vi "test.vi"() -> ()   [LabVIEW 2016]
uses:
  C:/Users/sciollalab/Documents/Brandeis-BNL/LabVIEW_Codes/BNLStaveAssembly-Blueprint/Bin/Aerotech.A3200.dll
  BNLStaveAssembly-Blueprint/Bin/Aerotech.A3200.dll
panel:
  in  "Axis Speeds":T1={"X [mm/s]"=10.0, "Y [mm/s]"=10.0, "Z [mm/s]"=10.0}
  out "Moving":bool
  in  "Program Errors":errorcluster
  out "XYZ Stage Control":refnum<k24>
  out "Stave origin":T2
  in  "XYZ Stage Frame: Coordinates for calibration":T3={"Stave origin"={"X [mm]"=-706.0, "Y [mm]"=140.5, "Z [mm]"=-13.5}, "Autofocus"={"X [mm]"=-686.0, "Y [mm]"=130.0, "Z [mm]"=-18.0}, "Calib Pattern"={"X [mm]"=-566.0, "Y [mm]"=39.26, "Z [mm]"=-22.0}}
  out "Current stage position [mm]":cluster{"X":dbl, "Y":dbl, "Z":dbl}
  in  "Update jog increment":bool
  in  "Jog step size":T2={"X [mm]"=0.1, "Y [mm]"=0.1, "Z [mm]"=0.1}
  in  "Backward":bool
  in  "Reset position":bool
  in  "Left":bool
  in  "Right":bool
  in  "Confirm position":bool
  in  "Forward":bool
  out "element":string
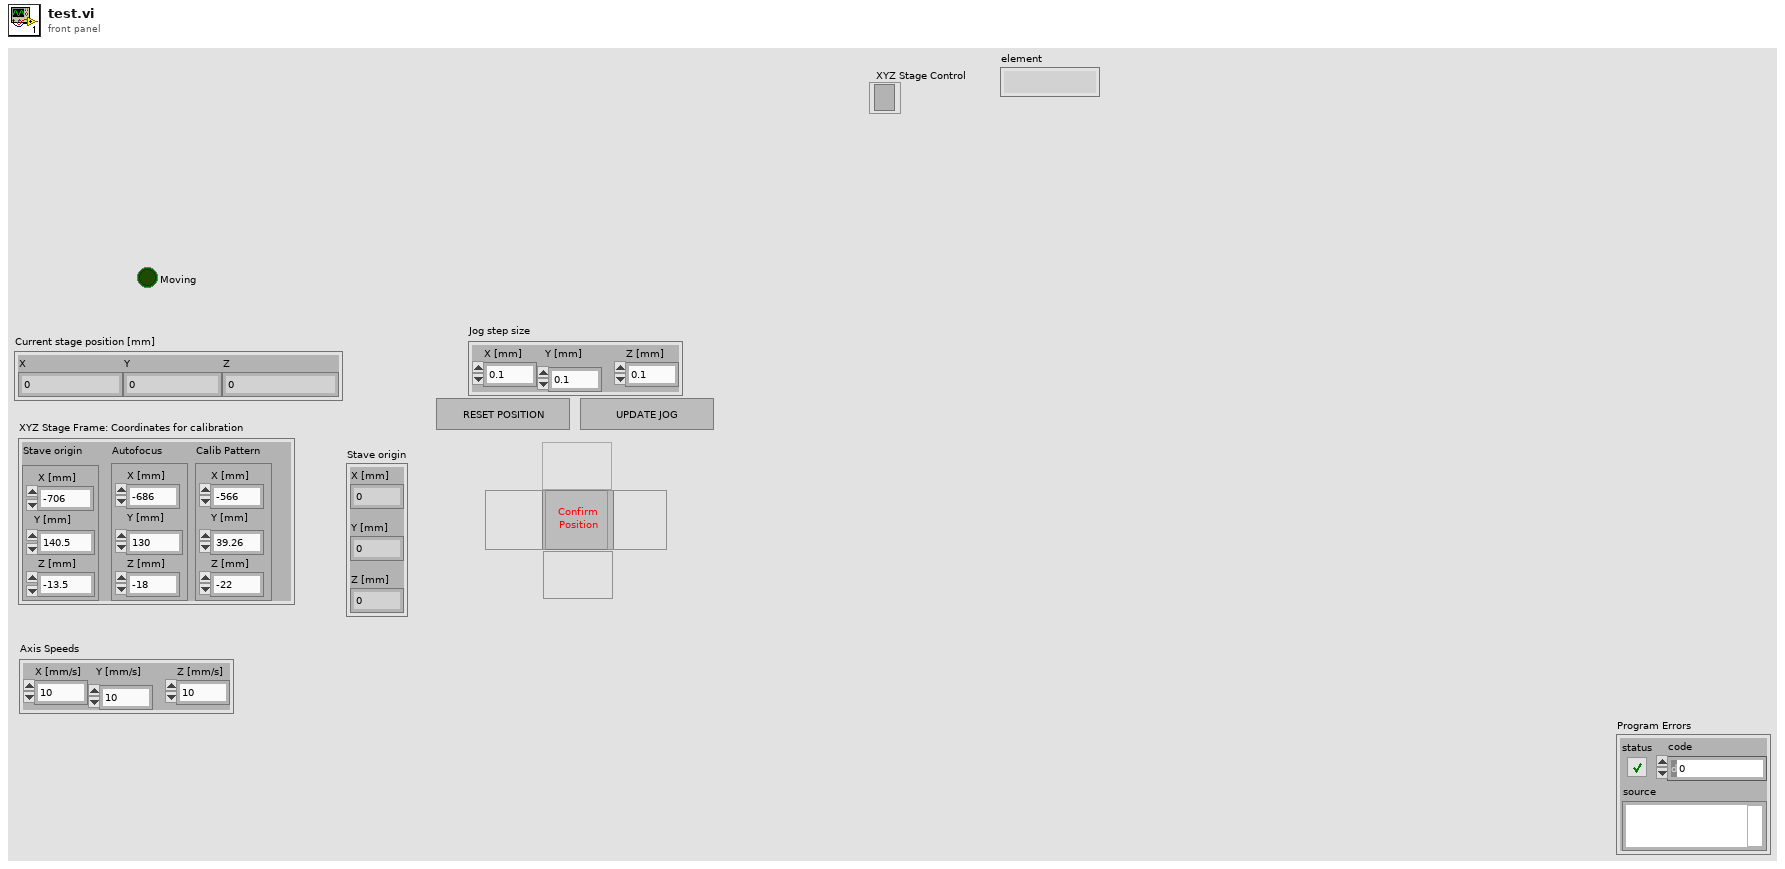
[diagram p1: front panel]
types:
  T1 = cluster{"X [mm/s]":dbl, "Y [mm/s]":dbl, "Z [mm/s]":dbl}
  T2 = cluster{"X [mm]":dbl, "Y [mm]":dbl, "Z [mm]":dbl}
  T3 = cluster{"Stave origin":cluster{"X [mm]":dbl, "Y [mm]":dbl, "Z [mm]":dbl}, "Autofocus":cluster{"X [mm]":dbl, "Y [mm]":dbl, "Z [mm]":dbl}, "Calib Pattern":cluster{"X [mm]":dbl, "Y [mm]":dbl, "Z [mm]":dbl}}
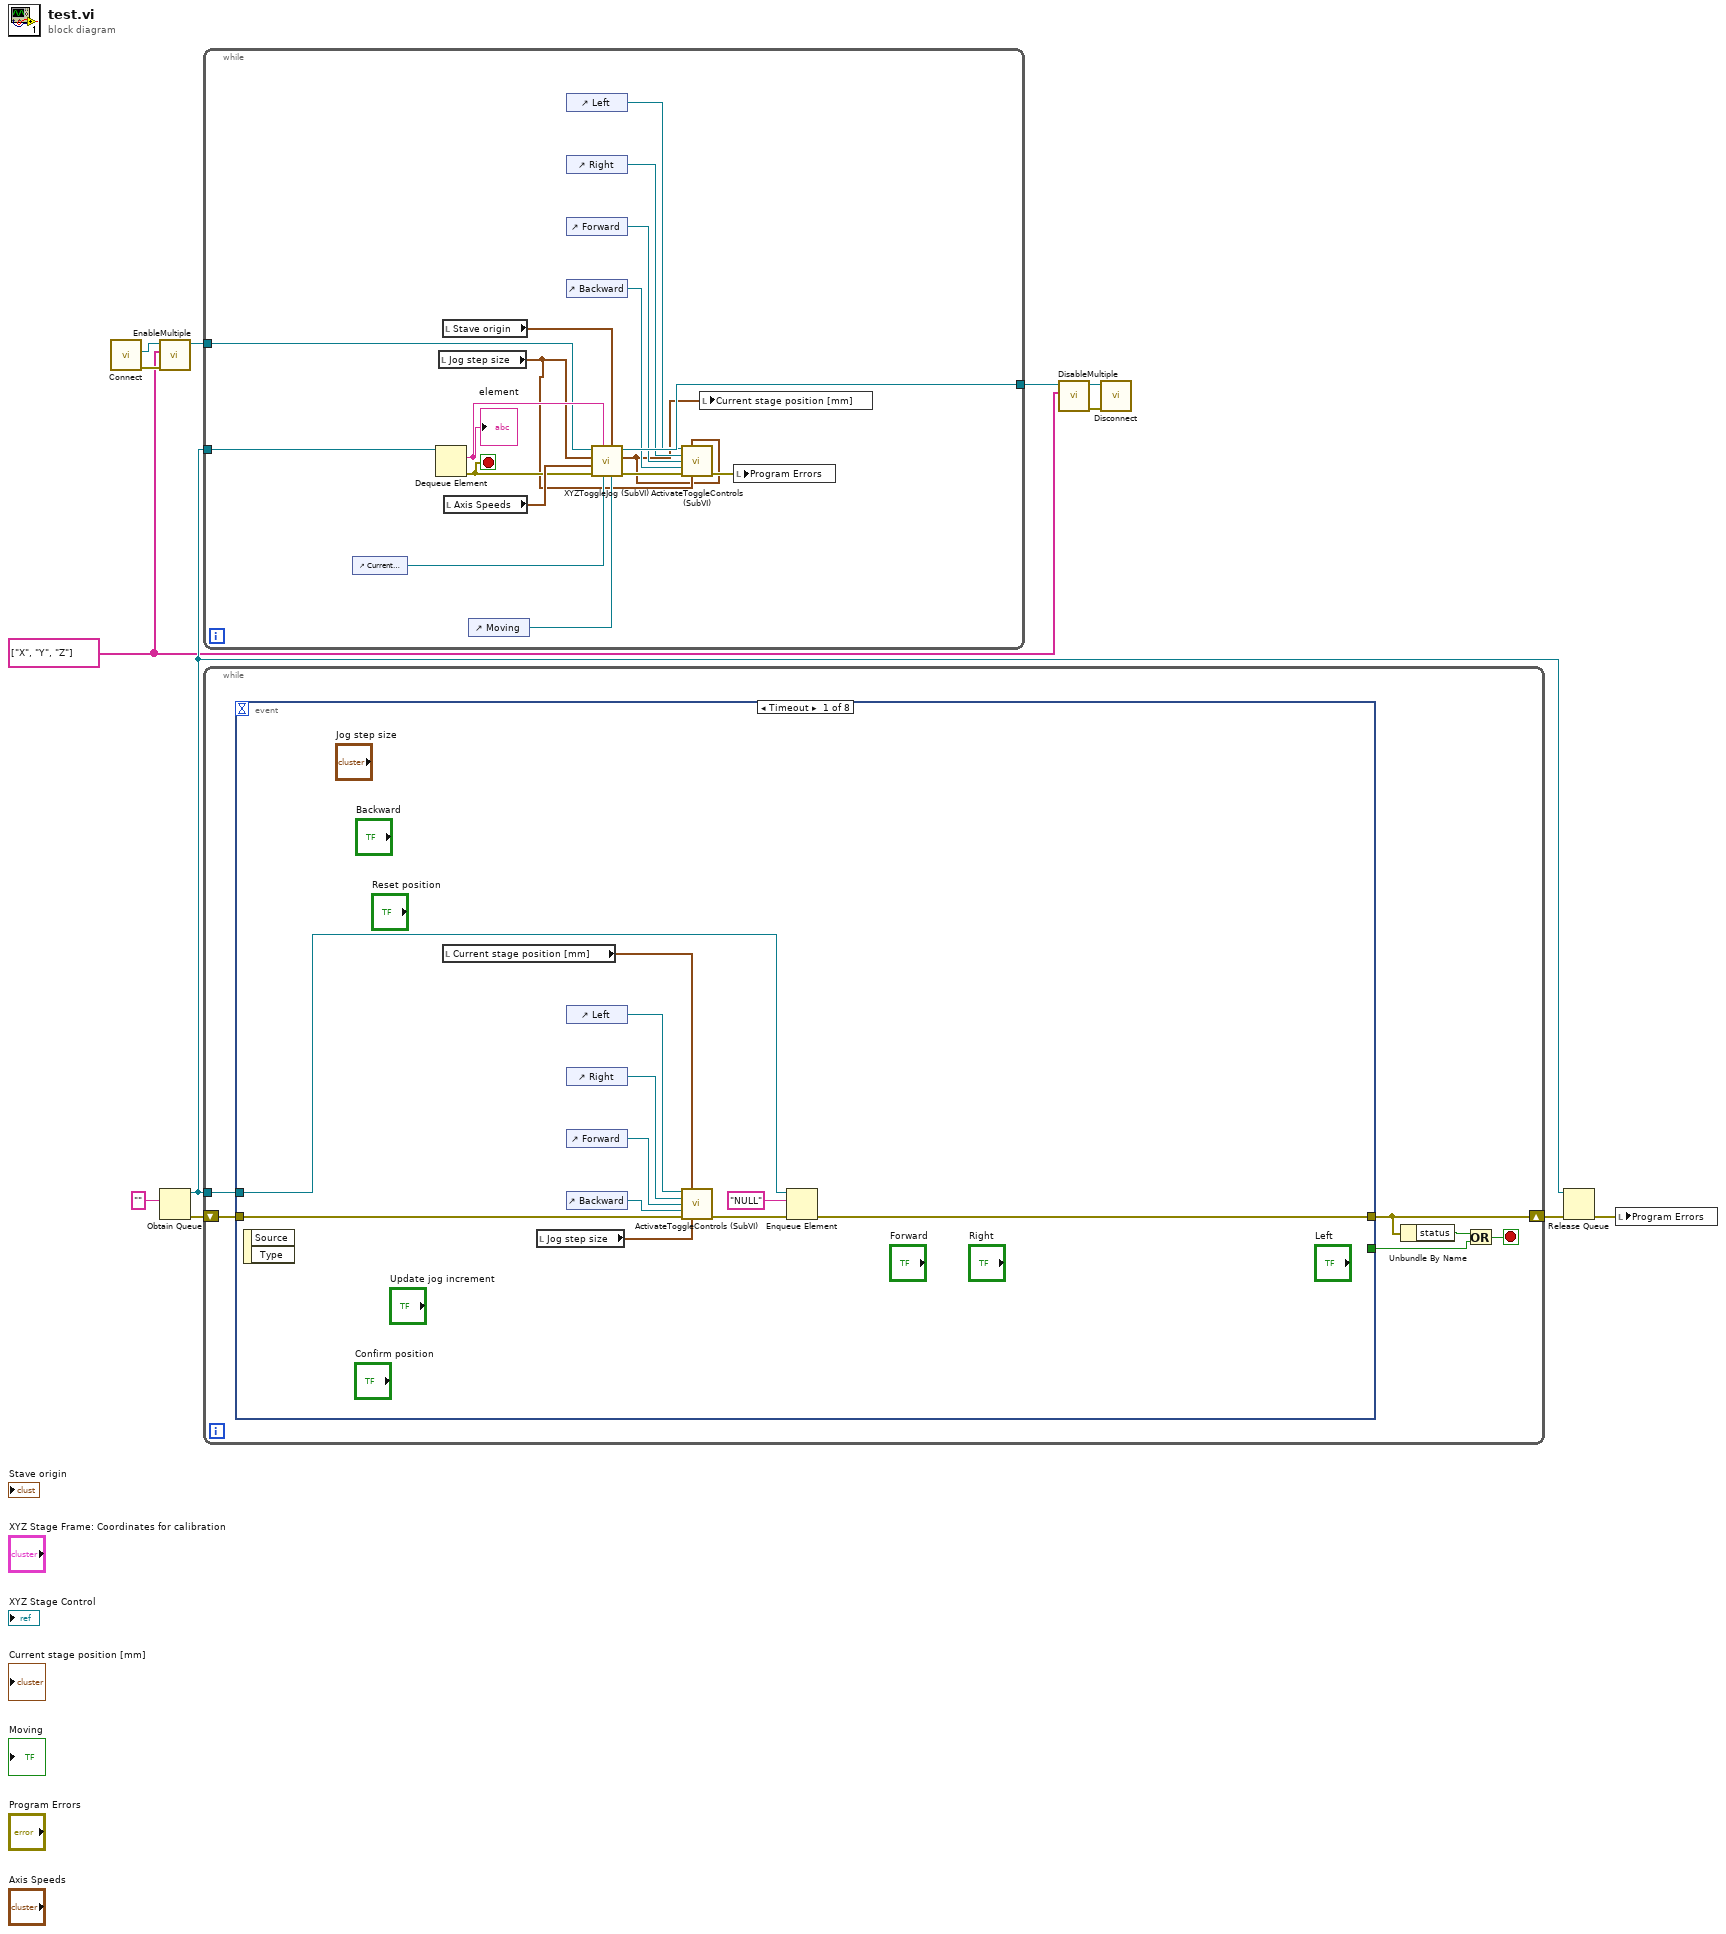
[diagram p0: block diagram]
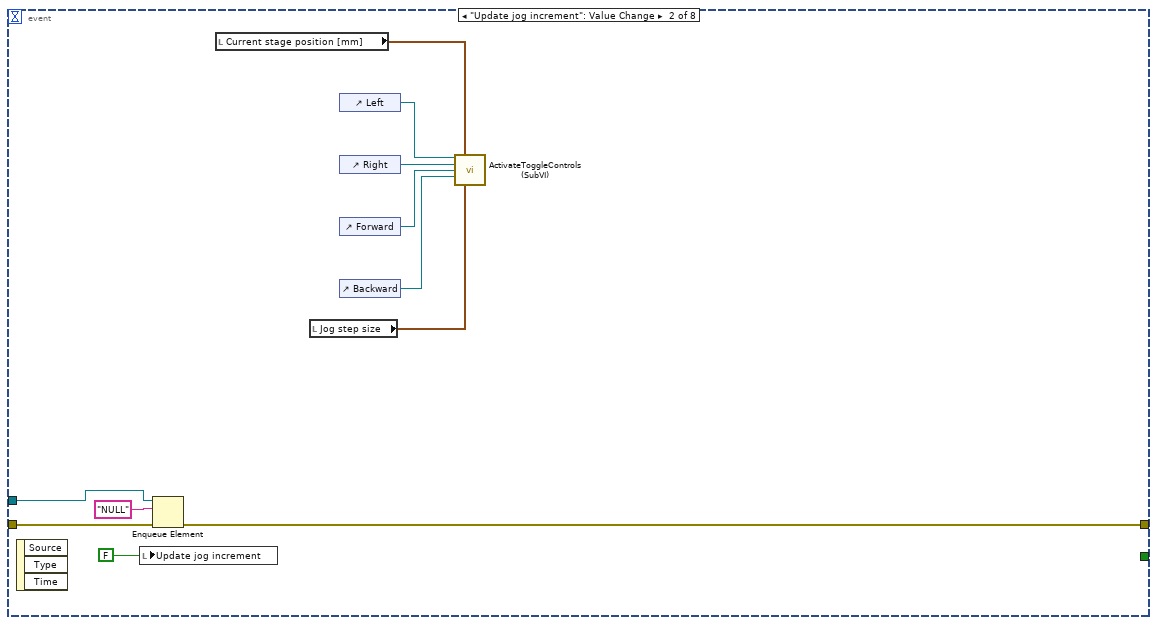
[diagram p2: hidden frame]
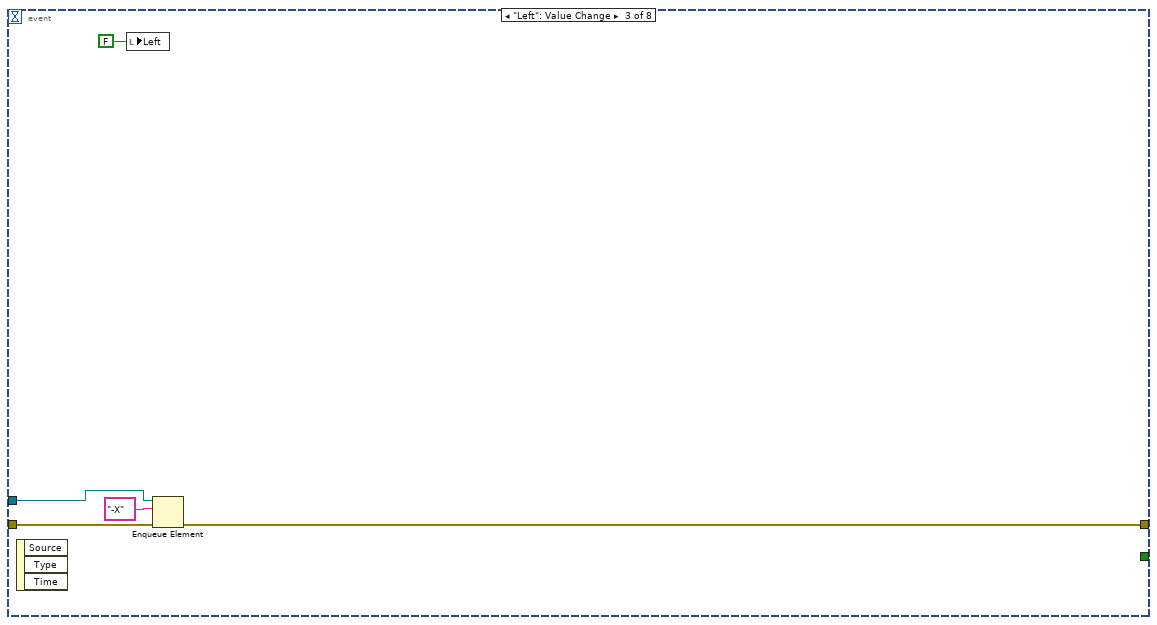
[diagram p3: hidden frame]
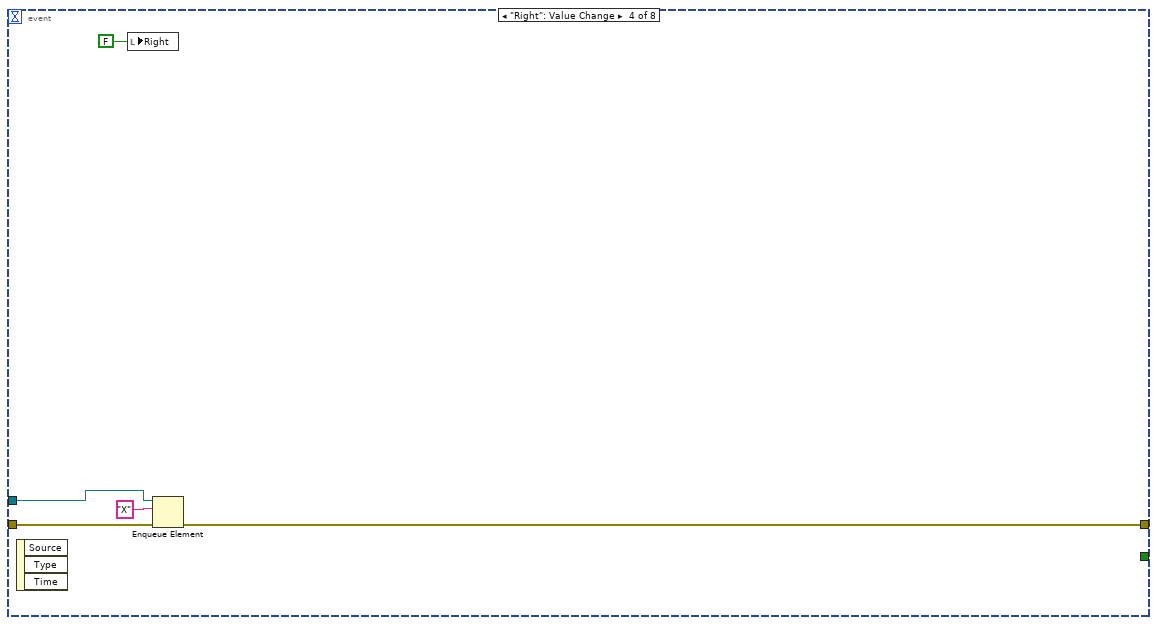
[diagram p4: hidden frame]
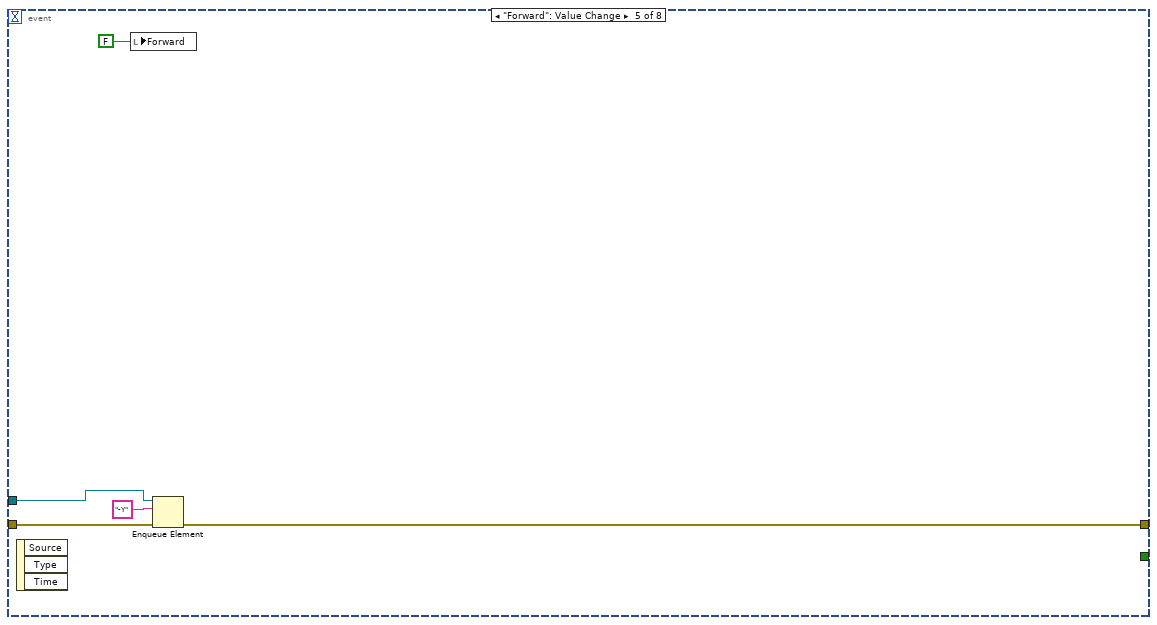
[diagram p5: hidden frame]
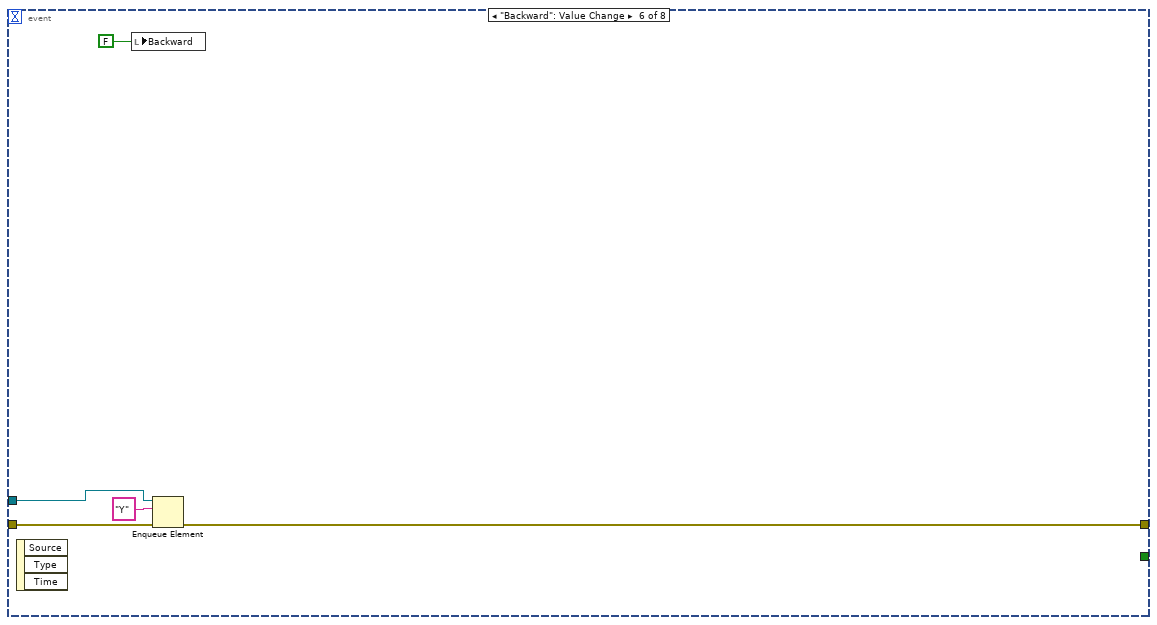
[diagram p6: hidden frame]
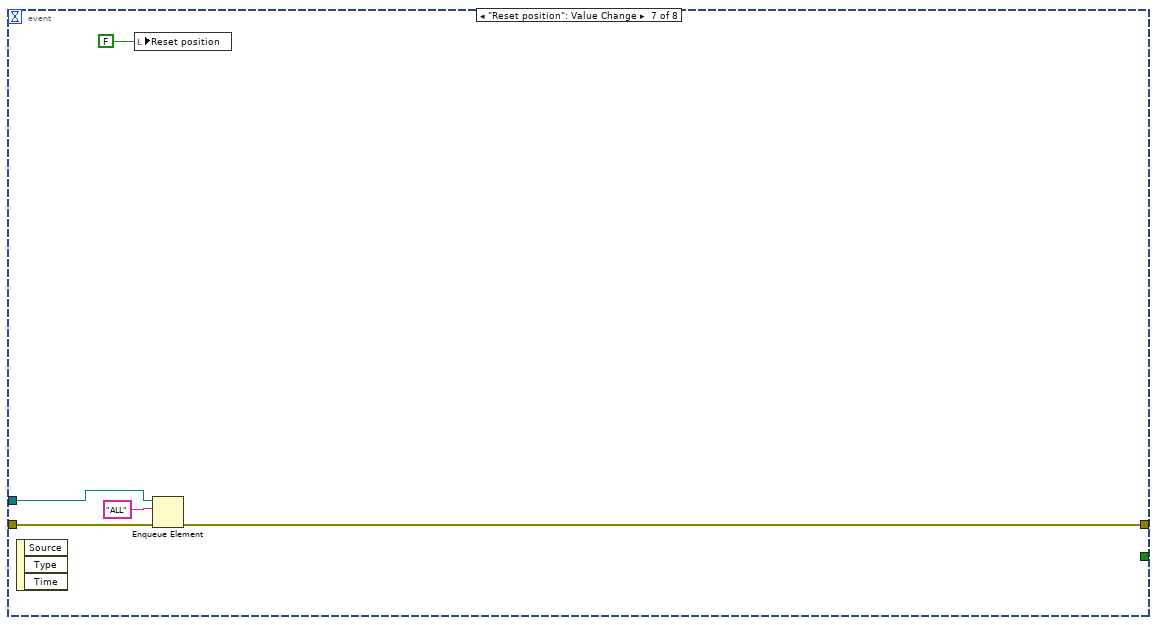
[diagram p7: hidden frame]
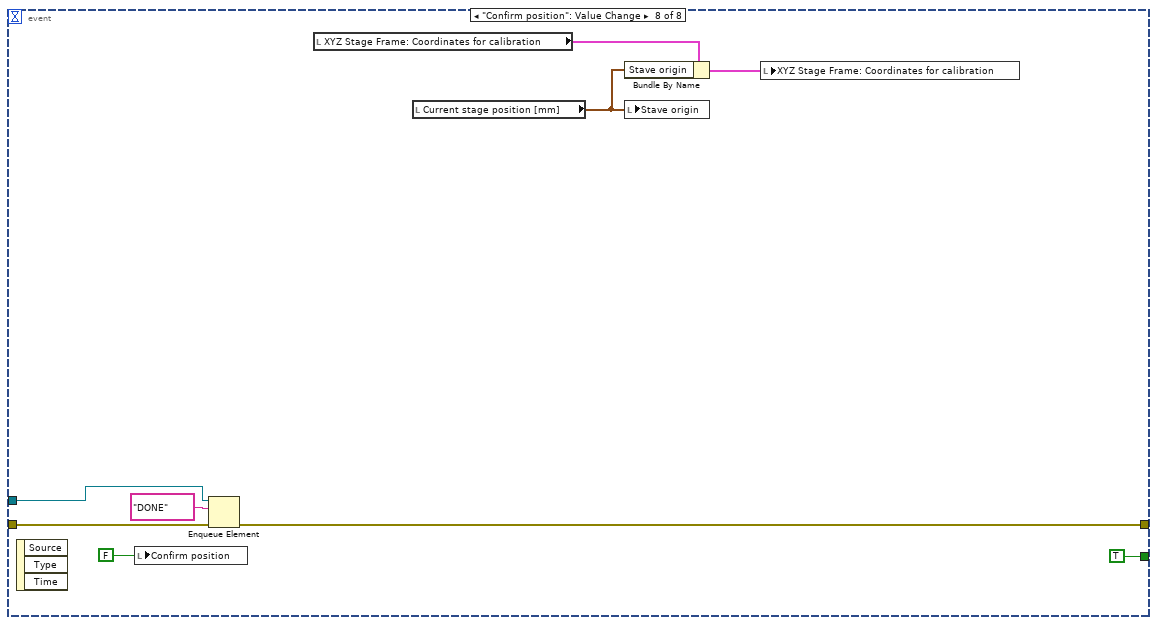
[diagram p8: hidden frame]
diagram:
  w2 = string[] ["X", "Y", "Z"] ("axis names")
  n1 = call "Connect.vi"() -> ("error out"=w7:errorcluster, "controller"=w6:refnum<k24>)  [unwired: 10 in]
  n2 = call "EnableMultiple.vi"("error in (no error)"=w7, "axis names"=w2, "controller in"=w6) -> ("controller out"=w1:refnum<k24>)  [unwired: 7 in, 1 out]
  n3 = Obtain Queue(element data type="") -> (queue out=w10:refnum<queue>, error out=w12:errorcluster)  [unwired: 4 in, 1 out]
  n4 = while {
    tunnel: w10 -> [w29]
    tunnel: [w23] -> w3
    tunnel: w1 -> [w22]
    stop <- w17 stop-if-true
    n5 = control-ref of="Current stage position [mm]"() -> (w26:refnum<vi>)
    n6 = Dequeue Element(queue=w29) -> (element=w24:string, error out=w17:errorcluster)  [unwired: 2 in, 2 out]
    "element" <- w24
    n7 = local read "Jog step size"() -> (w14:T2)
    n8 = local read "Stave origin"() -> (w28:T2)
    n9 = local read "Axis Speeds"() -> (w27:T1)
    n10 = control-ref of="Moving"() -> (w25:refnum<vi>)
    n11 = control-ref of="Left"() -> (w21:refnum<vi>)
    n12 = control-ref of="Right"() -> (w20:refnum<vi>)
    n13 = control-ref of="Forward"() -> (w19:refnum<vi>)
    n14 = control-ref of="Backward"() -> (w18:refnum<vi>)
    n15 = call "XYZToggleJog (SubVI).vi"("Moving"=w25, "Start location"=w28, "Stage position"=w26, "Motion direction"=w24, "error in (no error)"=w17, "Axis Speeds"=w27, "Jog step size"=w14, "Aerotech in"=w22) -> ("error out"=w16:errorcluster, "Current stage position [mm]"=w13:cluster{"X":dbl, "Y":dbl, "Z":dbl}, "Aerotech out"=w23:refnum<k24>)  [unwired: 1 out]
    n16 = call "ActivateToggleControls (SubVI).vi"("Left refnum"=w21, "Current stage position [mm]"=w13, "Right refnum"=w20, "Forward refnum"=w19, "Backward refnum"=w18, "error in (no error)"=w16, "Jog step size"=w14) -> ("error out"=w15:errorcluster)  [unwired: 8 in]
    n17 = local write "Current stage position [mm]"(w13) -> ()
    n18 = local write "Program Errors"(w15) -> ()
  }
  n19 = while {
    tunnel: w10 -> [w35]
    shift-right: [w33] -> w9
    shift-left: w12 -> [w34]
    stop <- w31 stop-if-true
    n20 = event shown="[0] Timeout" {
      selector: _ -> [_ _ _ _ _ _ _ _]
      dyn-events: _ -> [_ _ _ _ _ _ _ _]
      timeout: _ -> [_ _ _ _ _ _ _ _]
      tunnel: w35 -> [w39 w49 w60 w64 w71 w75 w81 w86]
      tunnel: w34 -> [w36 w48 w59 w66 w69 w74 w79 w83]
      tunnel: [w38 w47 w58 w65 w68 w73 w78 w84] -> w33
      tunnel: [_ _ _ _ _ _ _ TRUE] -> w30
      event Timeout {
        n21 = event-data() -> ()  [unwired: 1 in, 2 out]
        n22 = local read "Current stage position [mm]"() -> (w45:cluster{"X":dbl, "Y":dbl, "Z":dbl})
        n23 = local read "Jog step size"() -> (w46:T2)
        n24 = control-ref of="Left"() -> (w41:refnum<vi>)
        n25 = control-ref of="Right"() -> (w42:refnum<vi>)
        n26 = control-ref of="Forward"() -> (w43:refnum<vi>)
        n27 = control-ref of="Backward"() -> (w44:refnum<vi>)
        n28 = call "ActivateToggleControls (SubVI).vi"("Left refnum"=w41, "Current stage position [mm]"=w45, "Right refnum"=w42, "Forward refnum"=w43, "Backward refnum"=w44, "error in (no error)"=w36, "Jog step size"=w46) -> ("error out"=w37:errorcluster)  [unwired: 8 in]
        n29 = Enqueue Element(queue=w39, element="NULL", error in (no error)=w37) -> (error out=w38:errorcluster)  [unwired: 1 in, 2 out]
      }
      event "Update jog increment": Value Change {
        n30 = event-data() -> ()  [unwired: 1 in, 3 out]
        n31 = local write "Update jog increment"(FALSE ("Update jog increment")) -> ()
        n32 = Enqueue Element(queue=w49, element="NULL", error in (no error)=w48) -> (error out=w47:errorcluster)  [unwired: 1 in, 2 out]
        n33 = local read "Current stage position [mm]"() -> (w52:cluster{"X":dbl, "Y":dbl, "Z":dbl})
        n34 = local read "Jog step size"() -> (w53:T2)
        n35 = control-ref of="Left"() -> (w54:refnum<vi>)
        n36 = control-ref of="Right"() -> (w55:refnum<vi>)
        n37 = control-ref of="Forward"() -> (w56:refnum<vi>)
        n38 = control-ref of="Backward"() -> (w57:refnum<vi>)
        n39 = call "ActivateToggleControls (SubVI).vi"("Left refnum"=w54, "Current stage position [mm]"=w52, "Right refnum"=w55, "Forward refnum"=w56, "Backward refnum"=w57, "Jog step size"=w53) -> ()  [unwired: 9 in, 1 out]
      }
      event "Left": Value Change {
        n40 = event-data() -> ()  [unwired: 1 in, 3 out]
        n41 = local write "Left"(FALSE ("Left")) -> ()
        n42 = Enqueue Element(queue=w60, element="-X", error in (no error)=w59) -> (error out=w58:errorcluster)  [unwired: 1 in, 2 out]
      }
      event "Right": Value Change {
        n43 = event-data() -> ()  [unwired: 1 in, 3 out]
        n44 = local write "Right"(FALSE ("Left")) -> ()
        n45 = Enqueue Element(queue=w64, element="X", error in (no error)=w66) -> (error out=w65:errorcluster)  [unwired: 1 in, 2 out]
      }
      event "Forward": Value Change {
        n46 = event-data() -> ()  [unwired: 1 in, 3 out]
        n47 = local write "Forward"(FALSE ("Left")) -> ()
        n48 = Enqueue Element(queue=w71, element="-Y", error in (no error)=w69) -> (error out=w68:errorcluster)  [unwired: 1 in, 2 out]
      }
      event "Backward": Value Change {
        n49 = event-data() -> ()  [unwired: 1 in, 3 out]
        n50 = local write "Backward"(FALSE ("Left")) -> ()
        n51 = Enqueue Element(queue=w75, element="Y", error in (no error)=w74) -> (error out=w73:errorcluster)  [unwired: 1 in, 2 out]
      }
      event "Reset position": Value Change {
        n52 = event-data() -> ()  [unwired: 1 in, 3 out]
        n53 = local write "Reset position"(FALSE ("Reset position")) -> ()
        n54 = Enqueue Element(queue=w81, element="ALL", error in (no error)=w79) -> (error out=w78:errorcluster)  [unwired: 1 in, 2 out]
      }
      event "Confirm position": Value Change {
        n55 = event-data() -> ()  [unwired: 1 in, 3 out]
        n56 = local write "Confirm position"(FALSE ("Confirm position")) -> ()
        n57 = Enqueue Element(queue=w86, element="DONE", error in (no error)=w83) -> (error out=w84:errorcluster)  [unwired: 1 in, 2 out]
        n58 = local read "XYZ Stage Frame: Coordinates for calibration"() -> (w89:T3)
        n59 = local read "Current stage position [mm]"() -> (w88:cluster{"X":dbl, "Y":dbl, "Z":dbl})
        n60 = Bundle By Name(cluster=w89, "Stave origin"=w88) -> (w90:T3)
        n61 = local write "Stave origin"(w88) -> ()
        n62 = local write "XYZ Stage Frame: Coordinates for calibration"(w90) -> ()
      }
    }
    n63 = Unbundle By Name(w33) -> ("status"=w32:bool)
    n64 = Or(x=w32, y=w30) -> (x .or. y?=w31:bool)
  }
  n65 = call "DisableMultiple.vi"("axis names"=w2, "controller in"=w3) -> ("error out"=w5:errorcluster, "controller out"=w4:refnum<k24>)  [unwired: 8 in]
  n66 = call "Disconnect.vi"("error in (no error)"=w5, "controller"=w4) -> ()  [unwired: 9 in, 1 out]
  n67 = Release Queue(queue=w10, error in (no error)=w9) -> (error out=w8:errorcluster)  [unwired: 1 in, 2 out]
  n68 = local write "Program Errors"(w8) -> ()
